vi "VMI_check_cPI_set_up.vi"(11 "Delay Cluster":T1={"System no."=0, "Identification"="", "Device ID out"=0, "Postion / mm"=[], "SN out"="", "Movement Range"=[], "Conn. Axes"=[], "Target Position / mm"=50.0, "Velocity / mm s^-1"=0.15, "Set-up"=FALSE, "Moving"=FALSE, "Step Size / mm "=0.15, "Stage Number"=0, "Polling Time /ms"=0}) -> ()   [LabVIEW 2015]
uses:
  Type defs/PI_delay_settings.ctl
panel:
  out "error out":errorcluster
  in  "error in":errorcluster
  out "Delay Cluster 2":T1={"System no."=0, "Identification"="", "Device ID out"=0, "Postion / mm"=[], "SN out"="", "Movement Range"=[], "Conn. Axes"=[], "Target Position / mm"=50.0, "Velocity / mm s^-1"=0.15, "Set-up"=FALSE, "Moving"=FALSE, "Step Size / mm "=0.15, "Stage Number"=0, "Polling Time /ms"=0}
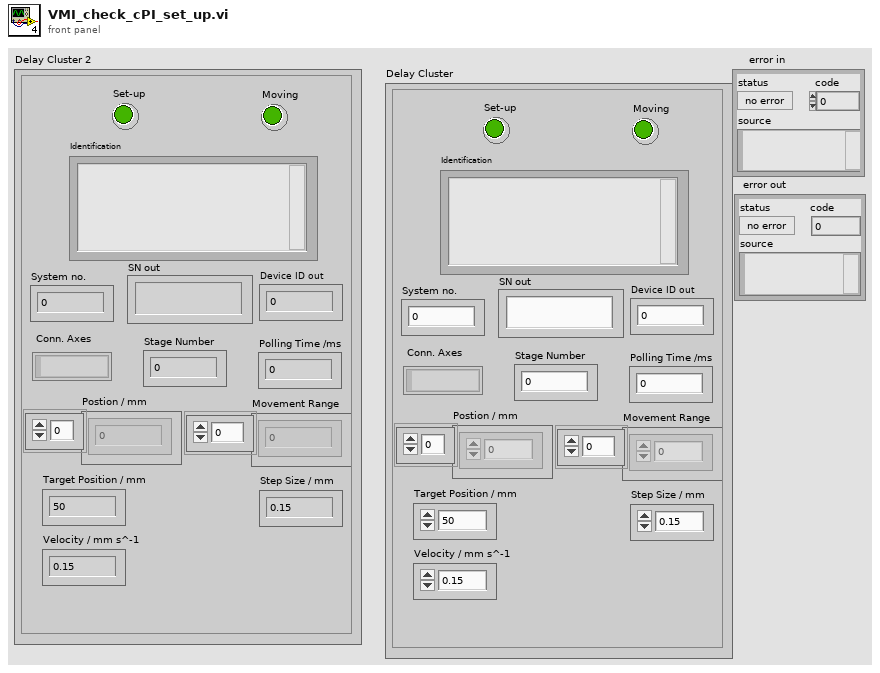
[diagram p1: front panel]
types:
  T1 = typedef "PI_delay_settings.ctl" = cluster{"System no.":i32, "Identification":string, "Device ID out":i32, "Postion / mm":dbl[], "SN out":string, "Movement Range":dbl[], "Conn. Axes":string[], "Target Position / mm":dbl, "Velocity / mm s^-1":dbl, "Set-up":bool, "Moving":bool, "Step Size / mm ":dbl, "Stage Number":i32, "Polling Time /ms":i32}
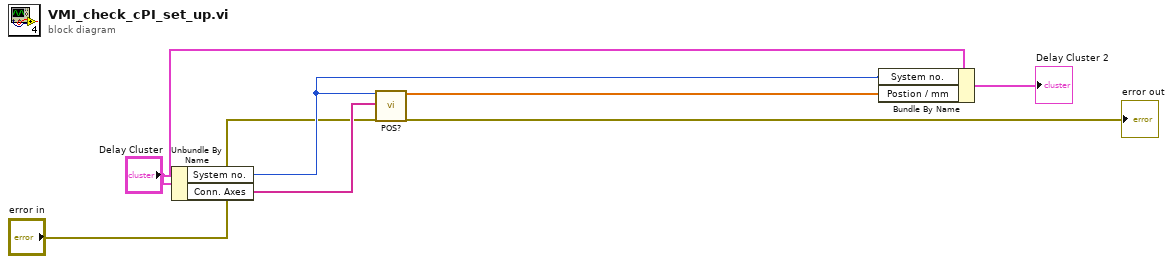
[diagram p0: block diagram]
diagram:
  n1 = Unbundle By Name("Delay Cluster") -> ("System no."=w4:i32, "Conn. Axes"=w7:string[])
  n2 = call "POS?.vi"("System no."=w4, "Axes to query"=w7, "error in"="error in") -> ("Position"=w3:dbl[], "error out"=→"error out":errorcluster)  [unwired: 2 in, 13 out]
  n3 = Bundle By Name(cluster="Delay Cluster", "System no."=w4, "Postion / mm"=w3) -> (→"Delay Cluster 2":T1)
